vi "saving plot.vi"() -> ()   [LabVIEW 2020]
uses:
  actor/data_handler/VDH-VNA_data_handler/VDH-VNA_data_handler/VDH-VNA_data_handler.lvclass
  actor/data_handler/VDH-VNA_data_handler/VDH-VNA_data_handler/VDH-VNA_data.ctl
  <vilib>/Utility/file.llb/Write Delimited Spreadsheet (DBL).vi
  <vilib>/Utility/file.llb/Read Delimited Spreadsheet (DBL).vi
  common/features/CF-common_features.lvlib
panel:
  out "File Path out":path
  out "deleted portion":dbl[][](array[numeric])
  out "number of rows":i32
  out "size(s)":i32[](array[numeric])
  out "array w/ subset deleted":dbl[][](array[numeric])
  out "all rows":dbl[][](array[numeric])
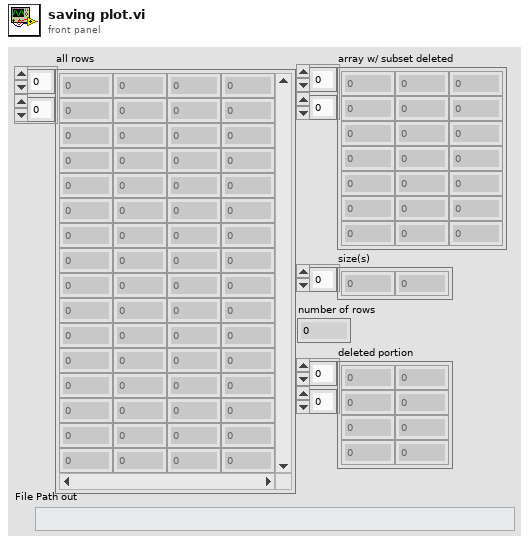
[diagram p1: front panel]
types:
  T1 = typedef "VDH-VNA_data_handler.lvlib/VDH-VNA_data_handler.lvclass/VDH-VNA_data.ctl" = cluster{"RP1":dbl[], "IP1":dbl[], "RP11":dbl[], "IP11":dbl[], "RP21":dbl[], "IP21":dbl[], "Frequency":u64[]}
  T2 = enum16{"open", "replace", "create", "open or create", "replace or create", "replace or create with confirmation"}
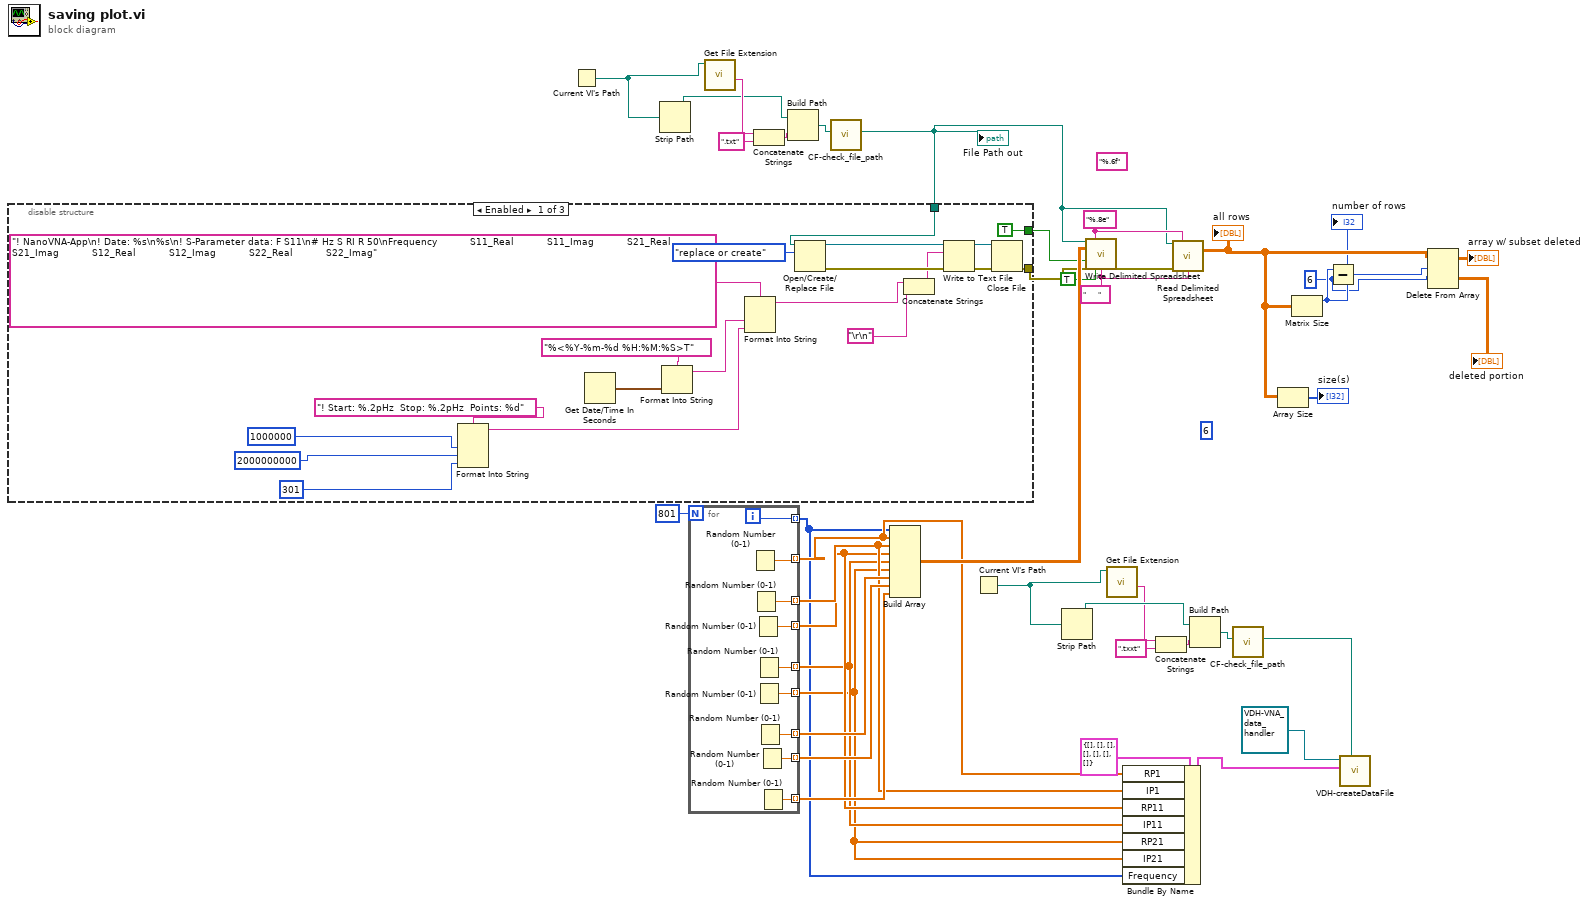
[diagram p0: block diagram]
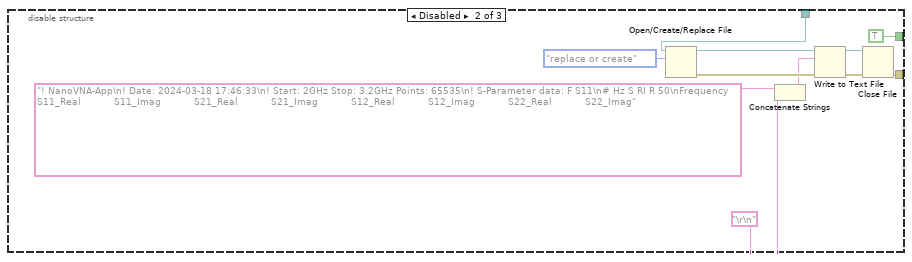
[diagram p2: hidden frame]
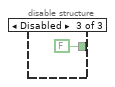
[diagram p3: hidden frame]
diagram:
  (unwired) "%.6f" ("format (%.3f)")
  w24 = "      " ("delimiter (\\t)")
  w23 = "%.8e" ("format (%.3f)")
  w26 = 6 ("y")
  (unwired) 6 ("start of read offset (chars.:0)")
  n1 = Current VI's Path() -> (path=w39:path)
  n2 = Strip Path(path=w39) -> (stripped path=w37:path)  [unwired: 1 out]
  n3 = for {
    N: 801 -> [_]
    tunnel: [w50] -> w6 mode=indexing
    tunnel: [w49] -> w5 mode=indexing
    tunnel: [w48] -> w1 mode=indexing
    tunnel: [w47] -> w4 mode=indexing
    tunnel: [w46] -> w3 mode=indexing
    tunnel: [w45] -> w2 mode=indexing
    tunnel: [w44] -> w20 mode=indexing
    tunnel: [w43] -> w19 mode=indexing
    tunnel: [w42] -> w18 mode=indexing
    i -> [w48]
    n4 = Random Number (0-1)() -> (number: 0 to 1=w50:dbl)
    n5 = Random Number (0-1)() -> (number: 0 to 1=w49:dbl)
    n6 = Random Number (0-1)() -> (number: 0 to 1=w47:dbl)
    n7 = Random Number (0-1)() -> (number: 0 to 1=w46:dbl)
    n8 = Random Number (0-1)() -> (number: 0 to 1=w45:dbl)
    n9 = Random Number (0-1)() -> (number: 0 to 1=w44:dbl)
    n10 = Random Number (0-1)() -> (number: 0 to 1=w43:dbl)
    n11 = Random Number (0-1)() -> (number: 0 to 1=w42:dbl)
  }
  n12 = call <vilib>:"Get File Extension.vi"("file"=w39) -> ("filename without extension"=w38:string)  [unwired: 6 in, 4 out]
  n13 = Concatenate Strings(w38, ".txt" ("string")) -> (w36:string)
  n14 = Build Path(base path=w37, name or relative path=w36) -> (appended path=w22:path)
  n15 = call "CF-check_file_path.vi"("File Path"=w22) -> ("File Path out"=w21:path)  [unwired: 10 in]
  "File Path out" <- w21
  n16 = disable-structure shown="Enabled" {
    disable-tunnel: [w66 w77 _] -> w34
    disable-tunnel: w21 -> [w64 w75 _]
    disable-tunnel: [TRUE ("append to file? (new file:F)") TRUE ("append to file? (new file:F)") FALSE ("append to file? (new file:F)")] -> w32
    frame Enabled {
      n17 = Format Into String(format string="! Start: %.2pHz  Stop: %.2pHz  Points: %d", u64 1000000 ("Measurement Settings.Start [hz]"), u64 2000000000 ("Measurement Settings.Start [hz]"), u64 301 ("Measurement Settings.Start [hz]")) -> (resulting string=w54:string)  [unwired: 2 in, 1 out]
      n18 = Get Date/Time In Seconds() -> (seconds since 1Jan1904=w58:timestamp)
      n19 = Format Into String(format string="%<%Y-%m-%d %H:%M:%S>T", w58) -> (resulting string=w56:string)  [unwired: 2 in, 1 out]
      n20 = Format Into String(format string="! NanoVNA-App\n! Date: %s\n%s\n! S-Parameter data: F S11\n# Hz S RI R 50\nFrequency           S11_Real           S11_Imag           S21_Real           S21_Imag           S12_Real           S12_Imag           S22_Real           S22_Imag" ("text"), w56, w54) -> (resulting string=w60:string)  [unwired: 2 in, 1 out]
      n21 = Open/Create/Replace File(file path (use dialog)=w64, operation (0:open)=T2."replace or create") -> (refnum out=w67:refnum<file>, error out=w68:errorcluster)  [unwired: 4 in, 1 out]
      n22 = Concatenate Strings(w60, "\r\n") -> (w61:string)
      n23 = Write to Text File(file (use dialog)=w67, text=w61, error in=w68) -> (refnum out=w69:refnum<file>, error out=w70:errorcluster)  [unwired: 1 in, 1 out]
      n24 = Close File(refnum=w69, error in=w70) -> (error out=w66:errorcluster)  [unwired: 1 out]
    }
    frame Disabled {
      n25 = Open/Create/Replace File(file path (use dialog)=w75, operation (0:open)=T2."replace or create") -> (refnum out=w78:refnum<file>, error out=w79:errorcluster)  [unwired: 4 in, 1 out]
      n26 = Concatenate Strings("! NanoVNA-App\n! Date: 2024-03-18 17:46:33\n! Start: 2GHz Stop: 3.2GHz Points: 65535\n! S-Parameter data: F S11\n# Hz S RI R 50\nFrequency           S11_Real           S11_Imag           S21_Real           S21_Imag           S12_Real           S12_Imag           S22_Real           S22_Imag" ("text"), "\r\n") -> (w71:string)
      n27 = Write to Text File(file (use dialog)=w78, text=w71, error in=w79) -> (refnum out=w80:refnum<file>, error out=w81:errorcluster)  [unwired: 1 in, 1 out]
      n28 = Close File(refnum=w80, error in=w81) -> (error out=w77:errorcluster)  [unwired: 1 out]
    }
    frame Disabled {
    }
  }
  n29 = Build Array(w1, w6, w5, w4, w3, w2, w20, w19, w18) -> (w40:dbl[][])
  n30 = Current VI's Path() -> (path=w10:path)
  n31 = Strip Path(path=w10) -> (stripped path=w12:path)  [unwired: 1 out]
  n32 = call-poly <vilib>:"Write Delimited Spreadsheet.vi"("file path (dialog if empty)"=w21, "format (%.3f)"=w23, "2D data"=w40, "append to file? (new file:F)"=w32, "error in (no error)"=w34, "transpose? (no:F)"=TRUE, "delimiter (\\t)"=w24) -> ("error out"=w33:errorcluster)  [unwired: 7 in, 1 out]
  n33 = call <vilib>:"Get File Extension.vi"("file"=w10) -> ("filename without extension"=w11:string)  [unwired: 6 in, 4 out]
  n34 = Bundle By Name(cluster=T1 {"RP1"=[], "IP1"=[], "RP11"=[], "IP11"=[], "RP21"=[], "IP21"=[], "Frequency"=[]} ("Data"), "RP1"=w6, "IP1"=w5, "RP11"=w4, "IP11"=w3, "RP21"=w2, "IP21"=w2, "Frequency"=w1) -> (w7:T1)
  n35 = Concatenate Strings(w11, ".txxt" ("string")) -> (w13:string)
  n36 = call-poly <vilib>:"Read Delimited Spreadsheet.vi"("file path (dialog if empty)"=w21, "format (%.3f)"=w23, "error in (no error)"=w33, "delimiter (\\t)"=w24) -> ("all rows"=w29:dbl[][])  [unwired: 6 in, 5 out]
  "all rows" <- w29
  n37 = Build Path(base path=w12, name or relative path=w13) -> (appended path=w15:path)
  n38 = call "CF-check_file_path.vi"("File Path"=w15) -> ("File Path out"=w9:path)  [unwired: 10 in]
  n39 = Array Size(array=w29) -> (size(s)=→"size(s)":i32[])
  n40 = Matrix Size(0:w29) -> (1:w28:i32)  [unwired: 1 out]
  "number of rows" <- w28
  n41 = Subtract(x=w28, y=w26) -> (x-y=w27:i32)
  n42 = call "VDH-createDataFile.vi"("file path (use dialog)"=w9, "Data"=w7, "VDH-VNA_data_handler in"=refnum<class "VDH-VNA_data_handler.lvclass"> refnum) -> ()  [unwired: 7 in, 2 out]
  n43 = Delete From Array(array=w29, length=w27, index (row)=w26) -> (deleted portion=→"deleted portion":dbl[][], array with subset deleted=→"array w/ subset deleted":dbl[][])  [unwired: 1 in]
